vi "Main.vi"(10 "Subpanel Ref":refnum<vi>, 11 "Module Admin":refnum<class "Delacor_lib_QMH_Module Admin.lvclass">) -> ()   [LabVIEW 2020, in "Disabled Property Panel.lvlib"]
doc: "This template is based off of the Queued Message Handler design pattern and the Queued Message Handler project template that ships with LabVIEW.\n\nThe main difference is that the queue is private to this module and communication between modules is performed via Broadcast and Request events.\n\nRequest events are wrapped in public API methods and are handled in the Event Handling Loop (EHL) of this VI. Any module can register for Broadcast events sent by this module. The EHL generates messages based on user interface actions.\n\nThe Message Handling Loop (MHL) processes messages generated by the EHL, or by other messages. The messages are string values, so new messages can be added easily to the Message Cases case structure in the MHL. Each message cluster can also provide an optional value for Message Data, which is a variant that can be converted to whatever message-specific data is required.\n_____\nBased on Delacor QMH Project Template 5.0.0.82."
uses:
  Disabled Property Panel.lvlib
  <vilib>/Delacor/Delacor QMH/Libraries/Module Admin_class/Delacor_lib_QMH_Module Admin.lvclass
  Module Data--cluster.ctl
  <vilib>/Delacor/Delacor QMH/Libraries/Message Queue_class/Delacor_lib_QMH_Message Queue.lvclass/Delacor_lib_QMH_Message Queue.ctl
  Stop Argument--cluster.ctl
  <vilib>/Delacor/Delacor QMH/Libraries/Module Admin_class/Delacor_lib_QMH_Module Admin.lvclass/Delacor_lib_QMH_Module Admin.ctl
  Initialize Property Value Argument--cluster.ctl
  <vilib>/Utility/miscctls.llb/LVPointTypeDef.ctl
  <vilib>/Delacor/Delacor QMH/Libraries/Message Queue_class/Delacor_lib_QMH_Enqueue Message (Single).vi
  <vilib>/Delacor/Delacor QMH/Libraries/Module Admin_class/Delacor_lib_QMH_Get External Launch.vi
  <vilib>/Utility/error.llb/Error Cluster From Error Code.vi
  <vilib>/ErrorRing/Error Ring.xnode
  <vilib>/Delacor/Delacor QMH/Libraries/Message Queue_class/Delacor_lib_QMH_Message Queue.lvclass
panel:
  in  "Disabled Property":T1(ring)
  in  "Simulate MHL Error":bool
  in  "Simulate EHL Error":bool
  out "error out":errorcluster
  out "Status":string
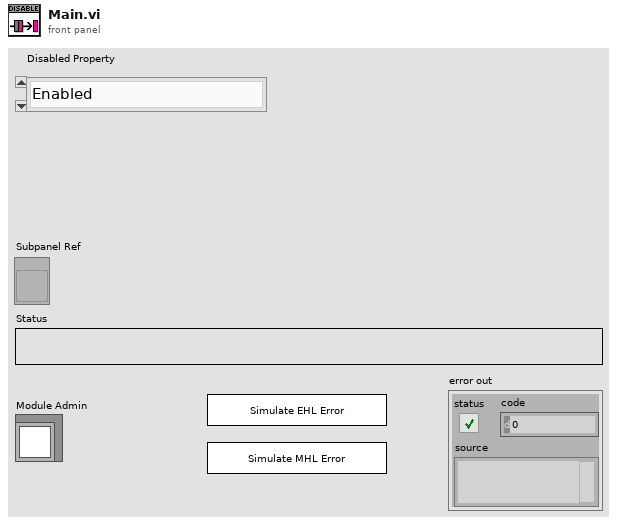
[diagram p1: front panel]
types:
  T1 = enum8{"Enabled", "Disabled", "Disabled and Grayed Out"}
  T2 = typedef "Disabled Property Panel.lvlib/Request Events--cluster.ctl" = cluster{"Stop Module":refnum<user-event>, "Show Panel":refnum<user-event>, "Hide Panel":refnum<user-event>, "Get Module Execution Status":refnum<user-event>, "Show Diagram":refnum<user-event>, "Initialize Property Value":refnum<user-event>}
  T3 = typedef "Disabled Property Panel.lvlib/Module Data--cluster.ctl" = cluster{"Status":string}
  T4 = enum32{"invalid lock state", "Not Locked", "Locked (No Password)", "Password-protected"}
  T5 = typedef "Disabled Property Panel.lvlib/Stop Argument--cluster.ctl" = cluster{"Origin":string, "Exit via Stop Module Req?":bool, "Wait for Module to stop?":bool}
  T6 = typedef "Disabled Property Panel.lvlib/Initialize Property Value Argument--cluster.ctl" = cluster{"Current Property Value":variant}
  T7 = typedef "LVPointTypeDef.ctl" = cluster{"Horizontal":i16, "Vertical":i16}
  T8 = cluster{"Property value":string, "Variant data":variant}
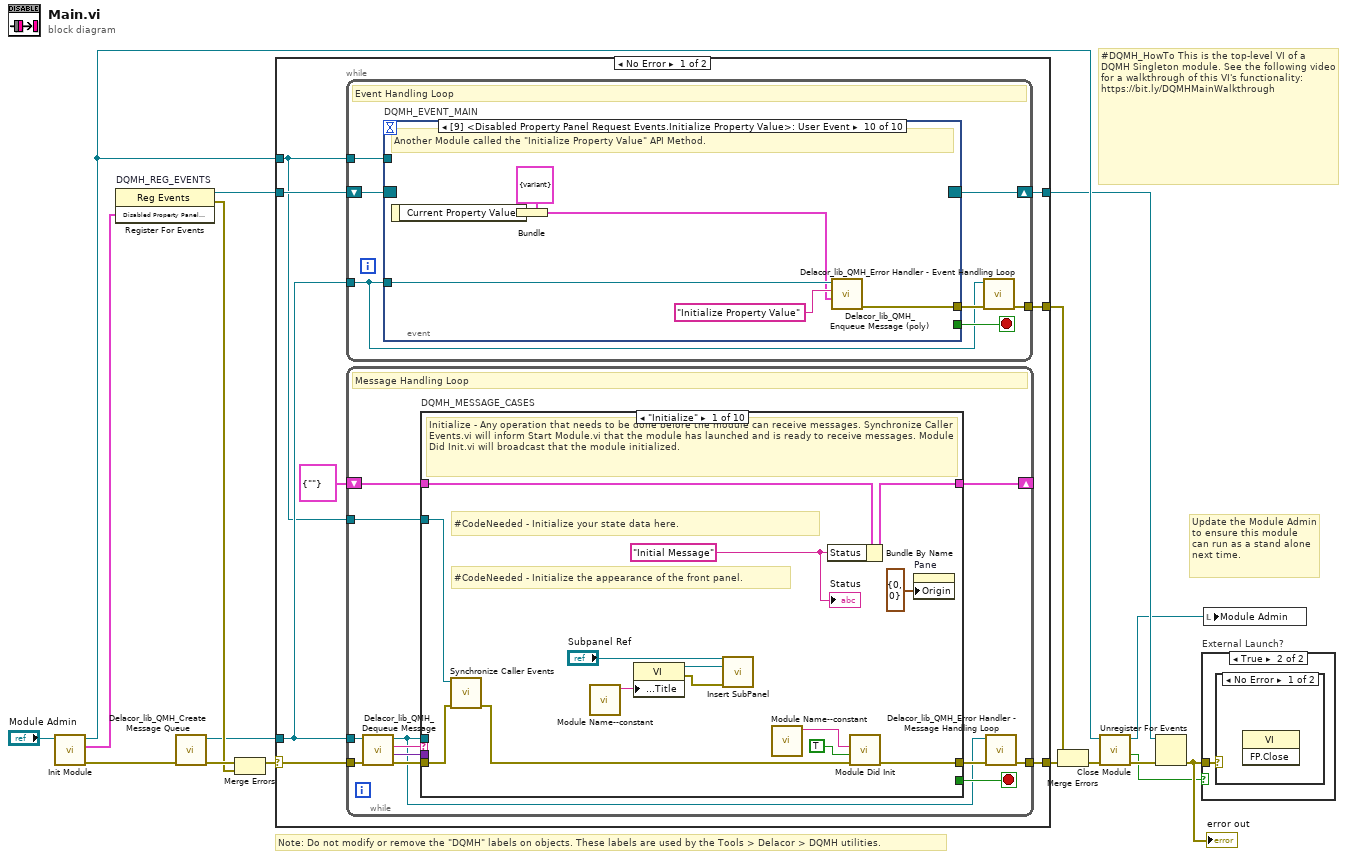
[diagram p0: block diagram]
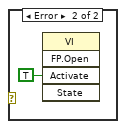
[diagram p3: hidden frame]
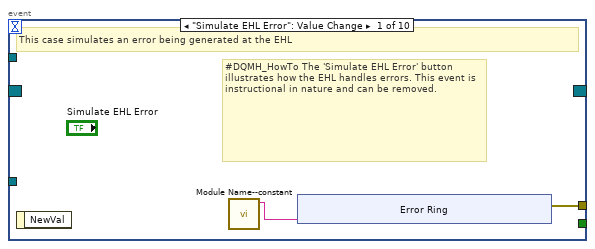
[diagram p4: hidden frame]
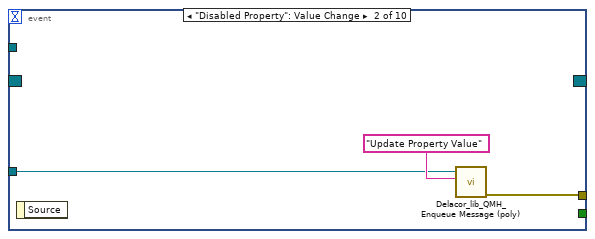
[diagram p5: hidden frame]
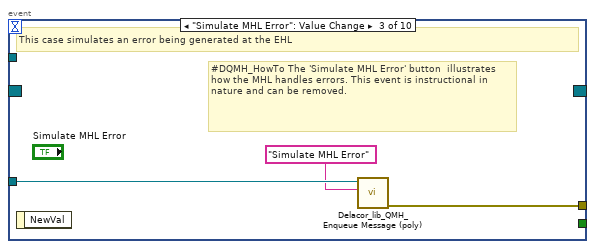
[diagram p6: hidden frame]
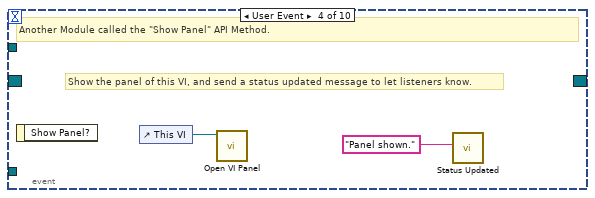
[diagram p7: hidden frame]
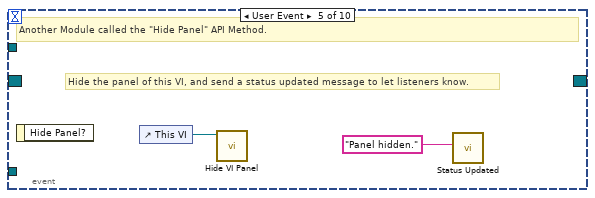
[diagram p8: hidden frame]
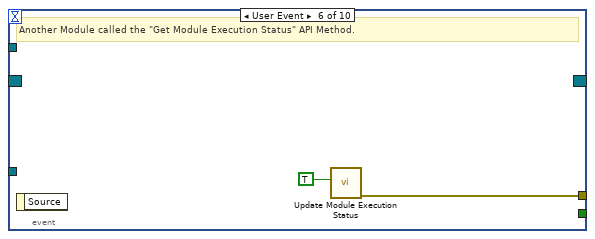
[diagram p9: hidden frame]
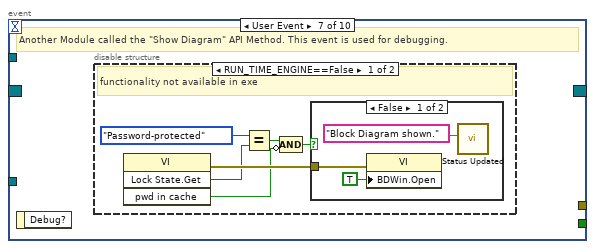
[diagram p10: hidden frame]
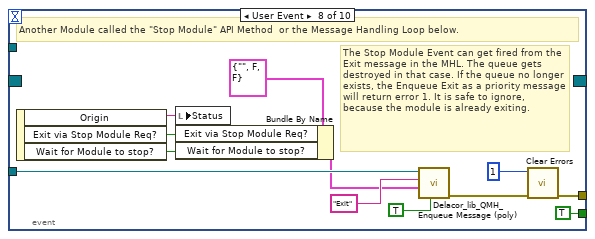
[diagram p13: hidden frame]
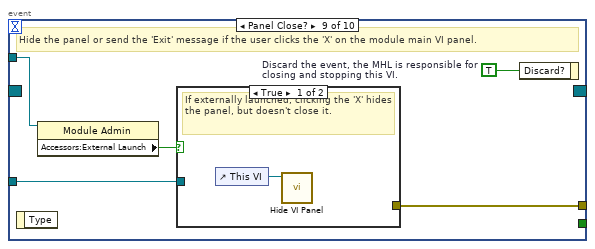
[diagram p14: hidden frame]
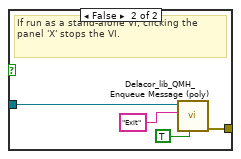
[diagram p15: hidden frame]
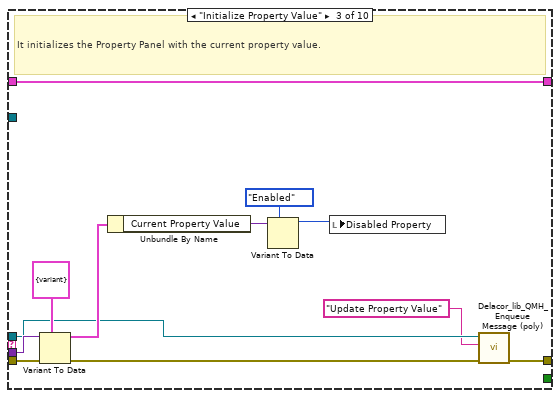
[diagram p17: hidden frame]
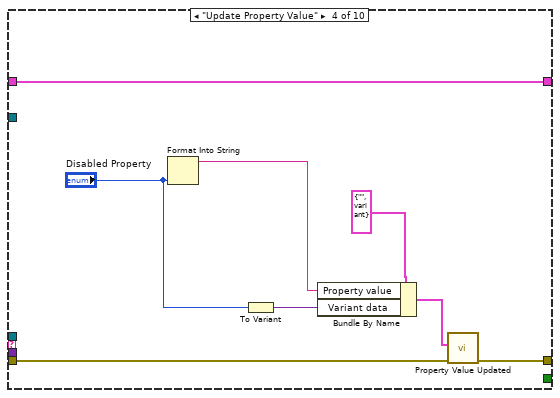
[diagram p18: hidden frame]
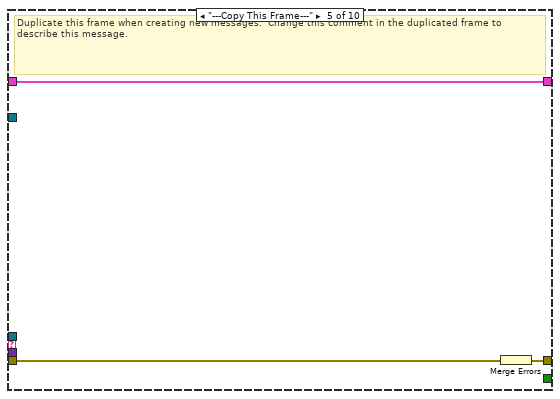
[diagram p19: hidden frame]
diagram:
  # "#DQMH_HowTo This is the top-level VI of a DQMH Singleton module. See the following video for a walkthrough of this VI's functionality: https://bit.ly/DQMHMainWalkthrough"
  # "Note: Do not modify or remove the \"DQMH\" labels on objects. These labels are used by the Tools > Delacor > DQMH utilities."
  # "Update the Module Admin to ensure this module can run as a stand alone next time."
  n1 = call "Init Module.vi"("Singleton Module Admin in"="Module Admin") -> ("error out"=w16:errorcluster, "Disabled Property Panel Request Events"=w5:T2, "Singleton Module Admin out"=w8:refnum<class "Delacor_lib_QMH_Module Admin.lvclass">)  [unwired: 8 in]
  n2 = register-events "DQMH_REG_EVENTS"(w5) -> (reference out=w6:refnum<event-registration>, error out=w9:errorcluster)  [unwired: 2 in]
  n3 = call <vilib>:"Delacor_lib_QMH_Create Message Queue.vi"("error in (no error)"=w16) -> ("error out"=w11:errorcluster, "Message Queue"=w4:refnum<class "Delacor_lib_QMH_Message Queue.lvclass">)  [unwired: 9 in]
  n4 = Merge Errors(w11, w9) -> (w10:errorcluster)
  n5 = case shown="No Error" w10 {
    selector: w10 -> [w23 w204]
    tunnel: [w25 w203] -> w17
    tunnel: [w22 w209] -> w7
    tunnel: w6 -> [w20 w209]
    tunnel: w4 -> [w19 w202]
    tunnel: [w24 _] -> w14
    tunnel: w8 -> [w18 w205]
    frame No Error {
      n6 = while {
        tunnel: w19 -> [w26]
        shift-right: [w29] -> w22
        shift-left: w20 -> [w30]
        tunnel: [w31] -> w24
        tunnel: w18 -> [w27]
        stop <- w28 stop-if-true
        # "Event Handling Loop"
        n7 = event "DQMH_EVENT_MAIN" shown="[9] <Disabled Property Panel Request Events.Initialize Property Value>: User Event" {
          selector: w30 -> [_ _ _ _ _ _ _ _ _ _]
          dyn-events: [_ _ _ _ _ _ _ _ _ _] -> w29
          timeout: _ -> [_ _ _ _ _ _ _ _ _ _]
          tunnel: [_ _ _ _ _ _ _ TRUE ("Discard?") _ _] -> w28
          tunnel: w26 -> [_ w43 w46 _ _ _ _ w70 w77 w90]
          tunnel: [w34 w42 w47 _ _ w53 _ w73 w79 w85] -> w32
          tunnel: w27 -> [_ _ _ _ _ _ _ _ w76 _]
          event "Simulate EHL Error": Value Change {
            # "#DQMH_HowTo The 'Simulate EHL Error' button  illustrates how the EHL handles errors. This event is instructional in nature and can be removed."
            # "This case simulates an error being generated at the EHL"
            n8 = event-data() -> ()  [unwired: 1 in, 1 out]
            n9 = call "Module Name--constant.vi"() -> ("Module Name"=w33:string)  [unwired: 11 in]
            n10 = xnode "Error Ring"("parameter 0"=w33) -> ("error out"=w34:errorcluster)
          }
          event "Disabled Property": Value Change {
            n11 = event-data() -> ()  [unwired: 1 in, 1 out]
            n12 = call-poly <vilib>:"Delacor_lib_QMH_Enqueue Message (poly).vi"("Message"="Update Property Value", "Message Queue in"=w43) -> ("error out"=w42:errorcluster)  [unwired: 8 in, 1 out]
          }
          event "Simulate MHL Error": Value Change {
            # "#DQMH_HowTo The 'Simulate MHL Error' button  illustrates how the MHL handles errors. This event is instructional in nature and can be removed."
            # "This case simulates an error being generated at the EHL"
            n13 = event-data() -> ()  [unwired: 1 in, 1 out]
            n14 = call-poly <vilib>:"Delacor_lib_QMH_Enqueue Message (poly).vi"("Message"="Simulate MHL Error", "Message Queue in"=w46) -> ("error out"=w47:errorcluster)  [unwired: 8 in, 1 out]
          }
          event User Event {
            # "Show the panel of this VI, and send a status updated message to let listeners know."
            # "Another Module called the \"Show Panel\" API Method."
            n15 = event-data() -> ()  [unwired: 1 in, 1 out]
            n16 = control-ref of="This VI"() -> (w49:refnum<vi>)
            n17 = call "Open VI Panel.vi"("VI"=w49) -> ()  [unwired: 10 in, 1 out]
            n18 = call "Status Updated.vi"("Status"="Panel shown." ("format string")) -> ()  [unwired: 10 in, 1 out]
          }
          event User Event {
            # "Hide the panel of this VI, and send a status updated message to let listeners know."
            # "Another Module called the \"Hide Panel\" API Method."
            n19 = event-data() -> ()  [unwired: 1 in, 1 out]
            n20 = control-ref of="This VI"() -> (w51:refnum<vi>)
            n21 = call "Hide VI Panel.vi"("VI"=w51) -> ()  [unwired: 10 in, 1 out]
            n22 = call "Status Updated.vi"("Status"="Panel hidden." ("format string")) -> ()  [unwired: 10 in, 1 out]
          }
          event User Event {
            # "Another Module called the \"Get Module Execution Status\" API Method."
            n23 = event-data() -> ()  [unwired: 1 in, 1 out]
            n24 = call "Update Module Execution Status.vi"("Running?"=TRUE) -> ("error out"=w53:errorcluster)  [unwired: 10 in]
          }
          event User Event {
            # "Another Module called the \"Show Diagram\" API Method. This event is used for debugging."
            n25 = event-data() -> ()  [unwired: 1 in, 1 out]
            n26 = disable-structure shown="RUN_TIME_ENGINE==False" {
              frame condition #0 (active) {
                # "functionality not available in exe"
                n27 = invoke class="VI" method="Lock State.Get"() -> (error out=w59:errorcluster, "Get Lock State"=w58:T4, "pwd in cache"=w55:bool)  [unwired: 4 in, 1 out]
                n28 = Equal?(x=T4."Password-protected", y=w58) -> (x = y?=w56:bool)
                n29 = Compound Arithmetic op=AND(w56, invert w55) -> (w54:bool)
                n30 = case shown="False" w54 {
                  tunnel: w59 -> [w62 _]
                  frame False {
                    n31 = property class="VI"(error in=w62, "BDWin.Open"=TRUE ("Block Diagram Window:Open")) -> ()  [unwired: 1 in, 2 out]
                    n32 = call "Status Updated.vi"("Status"="Block Diagram shown." ("format string")) -> ()  [unwired: 10 in, 1 out]
                  }
                  frame True {
                    # "Password-protected VI, and the password is not in the cache. Do not show the diagram."
                  }
                }
              }
              frame condition #1 {
              }
            }
          }
          event User Event {
            # "The Stop Module Event can get fired from the Exit message in the MHL. The queue gets destroyed in that case. If the queue no longer exists, the Enqueue Exit as a priority message will return error 1. It is safe to ignore, because the module is already exiting."
            # "Another Module called the \"Stop Module\" API Method  or the Message Handling Loop below."
            n33 = event-data() -> ("Origin"=w69:string, "Exit via Stop Module Req?"=w65:bool, "Wait for Module to stop?"=w64:bool)  [unwired: 1 in]
            n34 = local write "Status"(w69) -> ()
            n35 = Bundle By Name(cluster=T5 {"Origin"="", "Exit via Stop Module Req?"=FALSE, "Wait for Module to stop?"=FALSE} ("Stop Argument"), "Exit via Stop Module Req?"=w65, "Wait for Module to stop?"=w64) -> (w63:T5)
            n36 = call-poly <vilib>:"Delacor_lib_QMH_Enqueue Message (poly).vi"("Priority Message? (F)"=TRUE, "Message Data"=w63, "Message"="Exit", "Message Queue in"=w70) -> ("error out"=w74:errorcluster)  [unwired: 6 in, 1 out]
            n37 = call <vilib>:"Clear Errors.vi"("error in (no error)"=w74, "specific error code to clear (0: all)"=1) -> ("error out"=w73:errorcluster)  [unwired: 4 in, 1 out]
          }
          event Panel Close? {
            w78 = TRUE  # Discard the event, the MHL is responsible for closing and stopping this VI.
            # "Hide the panel or send the 'Exit' message if the user clicks the 'X' on the module main VI panel."
            n38 = event-data() -> ()  [unwired: 1 in, 1 out]
            n39 = property class="Module Admin"(reference=w76) -> ("Accessors:External Launch"=w75:bool)  [unwired: 1 in, 2 out]
            n40 = case shown="True" w75 {
              tunnel: w77 -> [_ w83]
              tunnel: [_ w84] -> w79
              frame True {
                # "If externally launched, clicking the 'X' hides the panel, but doesn't close it."
                n41 = control-ref of="This VI"() -> (w80:refnum<vi>)
                n42 = call "Hide VI Panel.vi"("VI"=w80) -> ()  [unwired: 10 in, 1 out]
              }
              frame False {
                # "If run as a stand-alone VI, clicking the panel 'X' stops the VI."
                n43 = call-poly <vilib>:"Delacor_lib_QMH_Enqueue Message (poly).vi"("Priority Message? (F)"=TRUE, "Message"="Exit", "Message Queue in"=w83) -> ("error out"=w84:errorcluster)  [unwired: 7 in, 1 out]
              }
            }
            n44 = event-data("Discard?"=w78) -> ()  [unwired: 1 in, 1 out]
          }
          event User Event {
            # "Another Module called the \"Initialize Property Value\" API Method."
            n45 = event-data() -> ("Current Property Value"=w86:variant)  [unwired: 1 in]
            n46 = Bundle(cluster=T6 {"Current Property Value"=variant} ("Initialize Property Value Argument"), "Current Property Value"=w86) -> (w87:T6)
            n47 = call-poly <vilib>:"Delacor_lib_QMH_Enqueue Message (poly).vi"("Message Data"=w87, "Message"="Initialize Property Value", "Message Queue in"=w90) -> ("error out"=w85:errorcluster)  [unwired: 7 in, 1 out]
          }
        }
        n48 = call-dynamic "Delacor_lib_QMH_Error Handler - Event Handling Loop.vi"("error in (no error)"=w32, "Message Queue in"=w26) -> ("dup error in"=w31:errorcluster)  [unwired: 8 in, 1 out]
      }
      n49 = while {
        tunnel: w19 -> [w93]
        shift-right: [w97] -> _
        shift-left: T3 {"Status"=""} ("Data Cluster") -> [w98]
        tunnel: w23 -> [w101]
        tunnel: [w99] -> w25
        tunnel: w18 -> [w91]
        stop <- w96 stop-if-true
        # "Message Handling Loop"
        n50 = call-dynamic "Delacor_lib_QMH_Dequeue Message.vi"("error in (no error)"=w101, "Message Queue in"=w93) -> ("error out"=w100:errorcluster, "Message Data"=w94:variant, "Message"=w95:string, "Message Queue out"=w92:refnum<class "Delacor_lib_QMH_Message Queue.lvclass">)  [unwired: 6 in]
        n51 = case "DQMH_MESSAGE_CASES" shown="\"Initialize\"" w95 {
          selector: w95 -> [_ _ _ _ _ _ _ _ _ w189]
          tunnel: w92 -> [_ _ w120 _ _ _ _ w159 w181 _]
          tunnel: w100 -> [w116 w118 w130 w137 w141 w143 w148 w166 w187 w191]
          tunnel: [w114 w118 w121 w136 w140 w143 w147 w162 w184 w192] -> w102
          tunnel: w98 -> [w111 w117 w129 w138 w139 w142 w145 w161 w180 w190]
          tunnel: [w110 w117 w129 w138 w139 w142 w145 w161 w180 w190] -> w97
          tunnel: [_ _ _ _ _ _ _ _ w179 _] -> w96
          tunnel: w94 -> [_ _ w128 _ _ _ _ w160 w178 _]
          tunnel: w91 -> [w112 _ _ _ _ _ _ w158 w173 _]
          frame "Initialize" {
            w106 = "Initial Message" ("Initial Message")
            # "#CodeNeeded - Initialize the appearance of the front panel."
            # "#CodeNeeded - Initialize your state data here."
            # "Initialize - Any operation that needs to be done before the module can receive messages. Synchronize Caller Events.vi will inform Start Module.vi that the module has launched and is ready to receive messages. Module Did Init.vi will broadcast that the module initialized."
            n52 = call "Synchronize Caller Events.vi"("error in (no error)"=w116, "Singleton Module Admin in"=w112) -> ("error out"=w115:errorcluster)  [unwired: 8 in, 1 out]
            n53 = call "Module Name--constant.vi"() -> ("Module Name"=w113:string)  [unwired: 11 in]
            n54 = property class="VI"("Front Panel.Title"=w113) -> (reference out=w105:refnum<vi>, error out=w104:errorcluster)  [unwired: 2 in]
            n55 = call <userlib>:"Insert SubPanel.vi"("error in (no error)"=w104, "VI Ref"=w105, "Subpanel Ref"="Subpanel Ref") -> ()  [unwired: 8 in, 1 out]
            n56 = call "Module Name--constant.vi"() -> ("Module Name"=w108:string)  [unwired: 11 in]
            n57 = Bundle By Name(cluster=w111, "Status"=w106) -> (w110:T3)
            n58 = call "Module Did Init.vi"("error in (no error)"=w115, "Initialized?"=TRUE, "Origin"=w108) -> ("error out"=w114:errorcluster)  [unwired: 8 in]
            n59 = property on="Pane" class="Pane"("Origin"=T7 {"Horizontal"=0, "Vertical"=0}) -> ()  [unwired: 2 in, 2 out]
            "Status" <- w106
          }
          frame "--- Module Specific ---" {
            # "Separator -- The following cases handle messages specific to this Module."
          }
          frame "Initialize Property Value" {
            # "It initializes the Property Panel with the current property value."
            n60 = Variant To Data(error in=w130, type=T6 {"Current Property Value"=variant} ("Initialize Property Value Argument"), Variant=w128) -> (data=w126:T6, error out=w122:errorcluster)
            n61 = Unbundle By Name(w126) -> ("Current Property Value"=w125:variant)
            n62 = Variant To Data(type=T1."Enabled" ("Disabled Property"), Variant=w125) -> (data=w123:T1)  [unwired: 1 in, 1 out]
            n63 = local write "Disabled Property"(w123) -> ()
            n64 = call-poly <vilib>:"Delacor_lib_QMH_Enqueue Message (poly).vi"("error in (no error)"=w122, "Message"="Update Property Value", "Message Queue in"=w120) -> ("error out"=w121:errorcluster)  [unwired: 7 in, 1 out]
          }
          frame "Update Property Value" {
            n65 = Format Into String("Disabled Property") -> (resulting string=w133:string)  [unwired: 3 in, 1 out]
            n66 = To Variant(anything="Disabled Property") -> (Variant=w131:variant)
            n67 = Bundle By Name(cluster=T8 {"Property value"="", "Variant data"=variant} ("Property data"), "Property value"=w133, "Variant data"=w131) -> (w134:T8)
            n68 = call "Property Value Updated.vi"("error in (no error)"=w137, "Property data"=w134) -> ("error out"=w136:errorcluster)  [unwired: 9 in]
          }
          frame "---Copy This Frame---" {
            # "Duplicate this frame when creating new messages.  Change this comment in the duplicated frame to describe this message."
            n69 = Merge Errors(w141) -> (w140:errorcluster)
          }
          frame "--- Exit and Error Handling---" {
            # "Separator - The following cases handle errors and exit messages."
          }
          frame "Simulate MHL Error" {
            # "#DQMH_HowTo The 'Simulate MHL Error' button  illustrates how the MHL handles errors. This event is instructional in nature and can be removed."
            # "Simulate an error occurring at the MHL"
            n70 = call "Module Name--constant.vi"() -> ("Module Name"=w144:string)  [unwired: 11 in]
            n71 = xnode "Error Ring"("parameter 0"=w144) -> ("error out"=w146:errorcluster)
            n72 = Merge Errors(w148, w146) -> (w147:errorcluster)
          }
          frame "Error" {
            # "#CodeRecommended - If you ever change the name of this \"Error\" message, you'll need to update the name in the Check Loop Error.vi as well."
            # "#CodeRecommended - If the module is running in standalone mode (External Launch = FALSE), this code will pop up an error dialog and call the 'Exit' message if an error occurs. Add more fine-grained error handling here."
            # "Error - Check the error message data and respond accordingly. This message is sent by the \"Error Handler\" VIs at the end of each loop in this application."
            n73 = property class="Module Admin"(reference=w158) -> ("Accessors:External Launch"=w157:bool)  [unwired: 1 in, 2 out]
            n74 = Variant To Data(error in=w166, type=errorcluster {"status"=FALSE, "code"=0, "source"=""} ("error constant"), Variant=w160) -> (data=w167:errorcluster, error out=w164:errorcluster)
            n75 = call "Module Name--constant.vi"() -> ("Module Name"=w156:string)  [unwired: 11 in]
            n76 = call "Error Reported.vi"("Additional Information"=w156, "Error"=w167) -> ()  [unwired: 9 in, 1 out]
            n77 = case shown="False" w157 {
              tunnel: [w172 _] -> w163
              tunnel: w159 -> [w170 _]
              tunnel: w167 -> [w171 _]
              frame False {
                # "If the module is running standalone, then pop up an error dialog and call the \"Exit\" message."
                n78 = call <vilib>:"Simple Error Handler.vi"("error in (no error)"=w171) -> ()  [unwired: 4 in, 5 out]
                n79 = call-poly <vilib>:"Delacor_lib_QMH_Enqueue Message (poly).vi"("Priority Message? (F)"=TRUE, "Message"="Exit", "Message Queue in"=w170) -> ("error out"=w172:errorcluster)  [unwired: 7 in, 1 out]
              }
              frame True {
                # "If the module was launched externally, calling the Error Reported broadcast VI is the only action performed by the \"Error\" message. The module's caller can then process the error appropriately."
              }
            }
            n80 = Merge Errors(w164, w163) -> (w162:errorcluster)
            n81 = local write "error out"(w162) -> ()
          }
          frame "Exit" {
            w177 = 91  # 91: not all Exit messages will have an argument
            w179 = TRUE  # Stop the VI
            # "Release the message queue reference"
            # "#CodeNeeded - Add any required cleanup code here"
            # "Exit - Exit the application."
            n82 = Variant To Data(error in=w187, type=T5 {"Origin"="", "Exit via Stop Module Req?"=FALSE, "Wait for Module to stop?"=FALSE} ("Stop Argument"), Variant=w178) -> (data=w175:T5, error out=w183:errorcluster)
            n83 = call <vilib>:"Clear Errors.vi"("error in (no error)"=w183, "specific error code to clear (0: all)"=w177) -> ("error out"=w186:errorcluster)  [unwired: 4 in, 1 out]
            n84 = control-ref of="This VI"() -> (w174:refnum<vi>)
            n85 = call-dynamic "Delacor_lib_QMH_Release Message Queue.vi"("error in (no error)"=w186, "Message Queue"=w181) -> ("error out"=w185:errorcluster)  [unwired: 9 in]
            n86 = call "Handle Exit.vi"("Stop Argument"=w175, "Admin in"=w173, "VI reference"=w174) -> ("error out"=w182:errorcluster)  [unwired: 7 in, 1 out]
            n87 = Merge Errors(w185, w182) -> (w184:errorcluster)
          }
          frame Default {
            # "'Default' case only runs if there is a message that isn't defined in any of the other cases.  Output a programming error."
            n88 = call "Module Name--constant.vi"() -> ("Module Name"=w188:string)  [unwired: 11 in]
            n89 = xnode "Error Ring"("parameter 0"=w189, "parameter 1"=w188) -> ("error out"=w193:errorcluster)
            n90 = Merge Errors(w191, w193) -> (w192:errorcluster)
          }
        }
        n91 = call-dynamic "Delacor_lib_QMH_Error Handler - Message Handling Loop.vi"("error in (no error)"=w102, "Message Queue in"=w92) -> ("dup error in"=w99:errorcluster)  [unwired: 8 in, 1 out]
      }
    }
    frame Error {
      # "Synchronize Caller Events.vi will inform Start Module.vi that the module has launched and will let the code calling Start Module.vi register for broadcasts and would permit the caller receive the broadcast that an error occurred at launch time."
      n92 = call-dynamic "Delacor_lib_QMH_Release Message Queue.vi"("error in (no error)"=w204, "Message Queue"=w202) -> ("error out"=w203:errorcluster)  [unwired: 9 in]
      n93 = call "Synchronize Caller Events.vi"("Singleton Module Admin in"=w205) -> ("error out"=w210:errorcluster)  [unwired: 9 in, 1 out]
      n94 = call "Module Name--constant.vi"() -> ("Module Name"=w208:string)  [unwired: 11 in]
      n95 = Format Into String(format string="An error occurred during initialization. %s is no longer running.", w208) -> (resulting string=w206:string)  [unwired: 2 in, 1 out]
      n96 = Merge Errors(w203, w210) -> (w211:errorcluster)
      n97 = call "Error Reported.vi"("Additional Information"=w206, "Error"=w211) -> ()  [unwired: 9 in, 1 out]
    }
  }
  n98 = Merge Errors(w14, w17) -> (w13:errorcluster)
  n99 = call "Close Module.vi"("error in (no error)"=w13, "Module Admin in"=w8) -> ("error out"=w15:errorcluster, "External Launch"=w1:bool, "Module Admin out"=w2:refnum<class "Delacor_lib_QMH_Module Admin.lvclass">)  [unwired: 7 in]
  n100 = Unregister For Events(event registration refnum=w7, error in=w15) -> (error out=w12:errorcluster)
  "error out" <- w12
  n101 = case "External Launch?" shown="True" w1 {
    tunnel: w12 -> [_ w212]
    frame False {
    }
    frame True {
      n102 = case shown="No Error" w212 {
        frame No Error {
          n103 = invoke class="VI" method="FP.Close"() -> ()  [unwired: 3 in, 3 out]
        }
        frame Error {
          n104 = invoke class="VI" method="FP.Open"("Activate"=TRUE ("Activate?")) -> ()  [unwired: 4 in, 5 out]
        }
      }
    }
  }
  n105 = local write "Module Admin"(w2) -> ()
